vi "Main.vi"(7 "sweep rate, /min":dbl=0.2, 8 "sweep to:":dbl=-0.5, 9 "sweep":T6(radio)=enum."time_sweep") -> ()   [LabVIEW 2017] (continued)
                      n3711 = Number To Decimal String(number=w4969) -> (decimal integer string=w4968:string)  [unwired: 1 in]
                      n3712 = GPIB Write(0:w4968, 1:"OUTP?2") -> (6:w4974:errorcluster)  [unwired: 3 in, 1 out]
                      n3713 = GPIB Read(0:w4968, 1:3200, 3:w4974) -> (5:w4972:string)  [unwired: 2 in, 2 out]
                      n3714 = Fract/Exp String To Number(string=w4972) -> (number=w4971:dbl)  [unwired: 3 in, 1 out]
                      n3715 = Build Array (concatenate)(w4976, w4971) -> (w4975:dbl[])
                    }
                  }
                  n3716 = property on="data" class="Arr (strict)"("Value"=w4966) -> ()  [unwired: 2 in, 2 out]
                }
                frame #10 {
                  # "check if in-phase\nsignal on lock-in 6 \nis to be measured"
                  n3717 = property on="data" class="Arr (strict)"() -> ("Value"=w4978:dbl[])  [unwired: 2 in, 2 out]
                  n3718 = local read "SR830_6_ip"() -> (w4977:bool)
                  n3719 = case shown="True" w4977 {
                    tunnel: w4978 -> [w4980 w4989]
                    tunnel: [w4980 w4988] -> w4979
                    frame False {
                      # "we are not measuring in phase signal on lock-in 6 (SR830_6_ip)"
                    }
                    frame True {
                      # "we are  measuring lock-in 6 in phase (SR830_6_ip)"
                      n3720 = local read "SR830_6"() -> (w4982:u8)
                      n3721 = Number To Decimal String(number=w4982) -> (decimal integer string=w4981:string)  [unwired: 1 in]
                      n3722 = GPIB Write(0:w4981, 1:"OUTR?1") -> (6:w4987:errorcluster)  [unwired: 3 in, 1 out]
                      n3723 = GPIB Read(0:w4981, 1:3200, 3:w4987) -> (5:w4985:string)  [unwired: 2 in, 2 out]
                      n3724 = Fract/Exp String To Number(string=w4985) -> (number=w4984:dbl)  [unwired: 3 in, 1 out]
                      n3725 = Build Array (concatenate)(w4989, w4984) -> (w4988:dbl[])
                    }
                  }
                  n3726 = property on="data" class="Arr (strict)"("Value"=w4979) -> ()  [unwired: 2 in, 2 out]
                }
                frame #11 {
                  # "check if out-of-phase\nsignal on lock-in 6 \nis to be measured"
                  n3727 = property on="data" class="Arr (strict)"() -> ("Value"=w4991:dbl[])  [unwired: 2 in, 2 out]
                  n3728 = local read "SR830_6_oop"() -> (w4990:bool)
                  n3729 = case shown="True" w4990 {
                    tunnel: w4991 -> [w4993 w5002]
                    tunnel: [w4993 w5001] -> w4992
                    frame False {
                      # "we are not measuring out of phase signal on lock-in 6 (SR830_6_oop)"
                    }
                    frame True {
                      # "we are  measuring lock-in 6, out of phase (SR830_6_oop)"
                      n3730 = local read "SR830_6"() -> (w4995:u8)
                      n3731 = Number To Decimal String(number=w4995) -> (decimal integer string=w4994:string)  [unwired: 1 in]
                      n3732 = GPIB Write(0:w4994, 1:"OUTR?2") -> (6:w5000:errorcluster)  [unwired: 3 in, 1 out]
                      n3733 = GPIB Read(0:w4994, 1:3200, 3:w5000) -> (5:w4998:string)  [unwired: 2 in, 2 out]
                      n3734 = Fract/Exp String To Number(string=w4998) -> (number=w4997:dbl)  [unwired: 3 in, 1 out]
                      n3735 = Build Array (concatenate)(w5002, w4997) -> (w5001:dbl[])
                    }
                  }
                  n3736 = property on="data" class="Arr (strict)"("Value"=w4992) -> ()  [unwired: 2 in, 2 out]
                }
                frame #12 {
                  # "check if in-phase\nsignal on lock-in 7 \nis to be measured"
                  n3737 = property on="data" class="Arr (strict)"() -> ("Value"=w5004:dbl[])  [unwired: 2 in, 2 out]
                  n3738 = local read "SR830_7_ip"() -> (w5003:bool)
                  n3739 = case shown="True" w5003 {
                    tunnel: w5004 -> [w5006 w5015]
                    tunnel: [w5006 w5014] -> w5005
                    frame False {
                    }
                    frame True {
                      # "we are  measuring lock-in 7 in phase (SR830_7_ip)"
                      n3740 = local read "SR830_7"() -> (w5008:u8)
                      n3741 = Number To Decimal String(number=w5008) -> (decimal integer string=w5007:string)  [unwired: 1 in]
                      n3742 = GPIB Write(0:w5007, 1:"OUTR?1") -> (6:w5013:errorcluster)  [unwired: 3 in, 1 out]
                      n3743 = GPIB Read(0:w5007, 1:3200, 3:w5013) -> (5:w5011:string)  [unwired: 2 in, 2 out]
                      n3744 = Fract/Exp String To Number(string=w5011) -> (number=w5010:dbl)  [unwired: 3 in, 1 out]
                      n3745 = Build Array (concatenate)(w5015, w5010) -> (w5014:dbl[])
                    }
                  }
                  n3746 = property on="data" class="Arr (strict)"("Value"=w5005) -> ()  [unwired: 2 in, 2 out]
                }
                frame #13 {
                  # "check if out-of-phase\nsignal on lock-in 7 \nis to be measured"
                  n3747 = property on="data" class="Arr (strict)"() -> ("Value"=w5017:dbl[])  [unwired: 2 in, 2 out]
                  n3748 = local read "SR830_7_oop"() -> (w5016:bool)
                  n3749 = case shown="True" w5016 {
                    tunnel: w5017 -> [w5019 w5028]
                    tunnel: [w5019 w5027] -> w5018
                    frame False {
                    }
                    frame True {
                      # "we are  measuring lock-in 7 out of phase (SR830_7_oop)"
                      n3750 = local read "SR830_7"() -> (w5021:u8)
                      n3751 = Number To Decimal String(number=w5021) -> (decimal integer string=w5020:string)  [unwired: 1 in]
                      n3752 = GPIB Write(0:w5020, 1:"OUTR?2") -> (6:w5026:errorcluster)  [unwired: 3 in, 1 out]
                      n3753 = GPIB Read(0:w5020, 1:3200, 3:w5026) -> (5:w5024:string)  [unwired: 2 in, 2 out]
                      n3754 = Fract/Exp String To Number(string=w5024) -> (number=w5023:dbl)  [unwired: 3 in, 1 out]
                      n3755 = Build Array (concatenate)(w5028, w5023) -> (w5027:dbl[])
                    }
                  }
                  n3756 = property on="data" class="Arr (strict)"("Value"=w5018) -> ()  [unwired: 2 in, 2 out]
                }
                frame #14 {
                  # "check if in-phase\nsignal on lock-in 8 \nis to be measured"
                  n3757 = property on="data" class="Arr (strict)"() -> ("Value"=w5030:dbl[])  [unwired: 2 in, 2 out]
                  n3758 = local read "SR830_8_ip"() -> (w5029:bool)
                  n3759 = case shown="True" w5029 {
                    tunnel: w5030 -> [w5032 w5041]
                    tunnel: [w5032 w5040] -> w5031
                    frame False {
                    }
                    frame True {
                      # "we are  measuring lock-in 8 in phase (SR830_8_ip)"
                      n3760 = local read "SR830_8"() -> (w5034:u8)
                      n3761 = Number To Decimal String(number=w5034) -> (decimal integer string=w5033:string)  [unwired: 1 in]
                      n3762 = GPIB Write(0:w5033, 1:"OUTR?1") -> (6:w5039:errorcluster)  [unwired: 3 in, 1 out]
                      n3763 = GPIB Read(0:w5033, 1:3200, 3:w5039) -> (5:w5037:string)  [unwired: 2 in, 2 out]
                      n3764 = Fract/Exp String To Number(string=w5037) -> (number=w5036:dbl)  [unwired: 3 in, 1 out]
                      n3765 = Build Array (concatenate)(w5041, w5036) -> (w5040:dbl[])
                    }
                  }
                  n3766 = property on="data" class="Arr (strict)"("Value"=w5031) -> ()  [unwired: 2 in, 2 out]
                }
                frame #15 {
                  # "check if out-of-phase\nsignal on lock-in 8 \nis to be measured"
                  n3767 = property on="data" class="Arr (strict)"() -> ("Value"=w5043:dbl[])  [unwired: 2 in, 2 out]
                  n3768 = local read "SR830_8_oop"() -> (w5042:bool)
                  n3769 = case shown="True" w5042 {
                    tunnel: w5043 -> [w5045 w5054]
                    tunnel: [w5045 w5053] -> w5044
                    frame False {
                    }
                    frame True {
                      # "we are  measuring lock-in 8 out of phase (SR830_8_oop)"
                      n3770 = local read "SR830_8"() -> (w5047:u8)
                      n3771 = Number To Decimal String(number=w5047) -> (decimal integer string=w5046:string)  [unwired: 1 in]
                      n3772 = GPIB Write(0:w5046, 1:"OUTR?2") -> (6:w5052:errorcluster)  [unwired: 3 in, 1 out]
                      n3773 = GPIB Read(0:w5046, 1:3200, 3:w5052) -> (5:w5050:string)  [unwired: 2 in, 2 out]
                      n3774 = Fract/Exp String To Number(string=w5050) -> (number=w5049:dbl)  [unwired: 3 in, 1 out]
                      n3775 = Build Array (concatenate)(w5054, w5049) -> (w5053:dbl[])
                    }
                  }
                  n3776 = property on="data" class="Arr (strict)"("Value"=w5044) -> ()  [unwired: 2 in, 2 out]
                }
                frame #16 {
                  # "Measure MFLI_V if \nit is checked"
                  n3777 = property on="MFLI_V1" class="Bool (strict)"() -> ("Value"=w5055:bool)  [unwired: 2 in, 2 out]
                  n3778 = property on="data" class="Arr (strict)"() -> ("Value"=w5057:dbl[])  [unwired: 2 in, 2 out]
                  n3779 = case shown="True" w5055 {
                    tunnel: w5057 -> [w5058 w5063]
                    tunnel: [w5058 w5062] -> w5056
                    frame False {
                      # "We are not recording Step Value if it is linetrace"
                    }
                    frame True {
                      n3780 = flat-sequence {
                        tunnel: [w5067] -> w5061
                        tunnel: [w5066] -> w5060
                        tunnel: [w5065] -> w5059
                        frame #0 {
                          n3781 = property on="HandleOut" class="Clust (strict)"() -> ("Value"=w5069:T5)  [unwired: 2 in, 2 out]
                          n3782 = call "MFLIcontrol.vi"("MFLI function"=MFLIcommand."measure XY on demod0", "handle in"=w5069) -> ("Demod Sample Out 2"=w5064:T22)  [unwired: 6 in, 3 out]
                          n3783 = Unbundle(w5064) -> ("X (Vrms)"=w5067:dbl, "Y (Vrms)"=w5066:dbl, "Freq (Hz)"=w5065:dbl)  [unwired: 6 out]
                        }
                      }
                      n3784 = Build Array (concatenate)(w5063, w5061, w5060, w5059) -> (w5062:dbl[])
                    }
                  }
                  n3785 = property on="data" class="Arr (strict)"("Value"=w5056) -> ()  [unwired: 2 in, 2 out]
                }
                frame #17 {
                  # "Measure MFLI_I if \nit is checked"
                  n3786 = property on="MFLI_I1" class="Bool (strict)"() -> ("Value"=w5070:bool)  [unwired: 2 in, 2 out]
                  n3787 = property on="data" class="Arr (strict)"() -> ("Value"=w5072:dbl[])  [unwired: 2 in, 2 out]
                  n3788 = case shown="True" w5070 {
                    tunnel: w5072 -> [w5073 w5078]
                    tunnel: [w5073 w5077] -> w5071
                    frame False {
                      # "We are not recording Step Value if it is linetrace"
                    }
                    frame True {
                      n3789 = flat-sequence {
                        tunnel: [w5081] -> w5076
                        tunnel: [w5080] -> w5075
                        tunnel: [w5079] -> w5074
                        frame #0 {
                          n3790 = property on="HandleOut" class="Clust (strict)"() -> ("Value"=w5084:T5)  [unwired: 2 in, 2 out]
                          n3791 = call "MFLIcontrol.vi"("MFLI function"=MFLIcommand."measure current", "handle in"=w5084) -> ("Demod Sample Out 3"=w5082:T22)  [unwired: 6 in, 3 out]
                          n3792 = Unbundle(w5082) -> ("X (Vrms)"=w5081:dbl, "Y (Vrms)"=w5080:dbl, "Freq (Hz)"=w5079:dbl)  [unwired: 6 out]
                        }
                      }
                      n3793 = Build Array (concatenate)(w5078, w5076, w5075, w5074) -> (w5077:dbl[])
                    }
                  }
                  n3794 = property on="data" class="Arr (strict)"("Value"=w5071) -> ()  [unwired: 2 in, 2 out]
                }
                frame #18 {
                  # "Measure MFLI_V if \nit is checked"
                  n3795 = local read "MFLI_V2"() -> (w5085:bool)
                  n3796 = property on="data" class="Arr (strict)"() -> ("Value"=w5087:dbl[])  [unwired: 2 in, 2 out]
                  n3797 = case shown="True" w5085 {
                    tunnel: w5087 -> [w5088 w5093]
                    tunnel: [w5088 w5092] -> w5086
                    frame False {
                    }
                    frame True {
                      n3798 = flat-sequence {
                        tunnel: [w5098] -> w5091
                        tunnel: [w5097] -> w5090
                        tunnel: [w5096] -> w5089
                        frame #0 {
                          n3799 = property on="Handle Out 2" class="Clust (strict)"() -> ("Value"=w5094:T5)  [unwired: 2 in, 2 out]
                          n3800 = call "MFLIcontrol.vi"("MFLI function"=MFLIcommand."measure XY on demod0", "handle in"=w5094) -> ("Demod Sample Out 2"=w5095:T22)  [unwired: 6 in, 3 out]
                          n3801 = Unbundle(w5095) -> ("X (Vrms)"=w5098:dbl, "Y (Vrms)"=w5097:dbl, "Freq (Hz)"=w5096:dbl)  [unwired: 6 out]
                        }
                      }
                      n3802 = Build Array (concatenate)(w5093, w5091, w5090, w5089) -> (w5092:dbl[])
                    }
                  }
                  n3803 = property on="data" class="Arr (strict)"("Value"=w5086) -> ()  [unwired: 2 in, 2 out]
                }
                frame #19 {
                  # "Measure MFLI_I if \nit is checked"
                  n3804 = local read "MFLI_I2"() -> (w5100:bool)
                  n3805 = property on="data" class="Arr (strict)"() -> ("Value"=w5102:dbl[])  [unwired: 2 in, 2 out]
                  n3806 = case shown="True" w5100 {
                    tunnel: w5102 -> [w5103 w5108]
                    tunnel: [w5103 w5107] -> w5101
                    frame False {
                    }
                    frame True {
                      n3807 = flat-sequence {
                        tunnel: [w5113] -> w5106
                        tunnel: [w5112] -> w5105
                        tunnel: [w5111] -> w5104
                        frame #0 {
                          n3808 = property on="Handle Out 2" class="Clust (strict)"() -> ("Value"=w5110:T5)  [unwired: 2 in, 2 out]
                          n3809 = call "MFLIcontrol.vi"("MFLI function"=MFLIcommand."measure current", "handle in"=w5110) -> ("Demod Sample Out 3"=w5109:T22)  [unwired: 6 in, 3 out]
                          n3810 = Unbundle(w5109) -> ("X (Vrms)"=w5113:dbl, "Y (Vrms)"=w5112:dbl, "Freq (Hz)"=w5111:dbl)  [unwired: 6 out]
                        }
                      }
                      n3811 = Build Array (concatenate)(w5108, w5106, w5105, w5104) -> (w5107:dbl[])
                    }
                  }
                  n3812 = property on="data" class="Arr (strict)"("Value"=w5101) -> ()  [unwired: 2 in, 2 out]
                }
                frame #20 {
                  # "check if voltage \non 2400 SouceMeter 1\nis to be measured"
                  n3813 = property on="data" class="Arr (strict)"() -> ("Value"=w5116:dbl[])  [unwired: 2 in, 2 out]
                  n3814 = local read "2400 1 meas v"() -> (w5115:bool)
                  n3815 = case shown="True" w5115 {
                    tunnel: w5116 -> [w5118 w5129]
                    tunnel: [w5118 w5128] -> w5117
                    frame False {
                      # "we are not measuring 2400 1, voltage (2400_1_v)"
                    }
                    frame True {
                      # "we are  measuring 2400 1, voltage (2400_1_v)"
                      n3816 = local read "2400 1 addr"() -> (w5123:u8)
                      n3817 = Number To Decimal String(number=w5123) -> (decimal integer string=w5122:string)  [unwired: 1 in]
                      n3818 = GPIB Write(0:w5122, 1:":READ?") -> (6:w5127:errorcluster)  [unwired: 3 in, 1 out]
                      n3819 = GPIB Read(0:w5122, 1:3200, 3:w5127) -> (5:w5120:string)  [unwired: 2 in, 2 out]
                      n3820 = String Subset(string=w5120, length (rest)=13) -> (substring=w5119:string)  [unwired: 1 in]
                      n3821 = Fract/Exp String To Number(string=w5119) -> (number=w5125:dbl)  [unwired: 3 in, 1 out]
                      n3822 = Build Array (concatenate)(w5129, w5125) -> (w5128:dbl[])
                    }
                  }
                  n3823 = property on="data" class="Arr (strict)"("Value"=w5117) -> ()  [unwired: 2 in, 2 out]
                }
                frame #21 {
                  # "check if current \non 2400 SouceMeter 1\nis to be measured"
                  n3824 = property on="data" class="Arr (strict)"() -> ("Value"=w5131:dbl[])  [unwired: 2 in, 2 out]
                  n3825 = local read "2400 1 meas i"() -> (w5130:bool)
                  n3826 = case shown="True" w5130 {
                    tunnel: w5131 -> [w5133 w5145]
                    tunnel: [w5133 w5144] -> w5132
                    frame False {
                      # "we are not measuring 2400 1, current (2400_1_i)"
                    }
                    frame True {
                      # "we are  measuring 2400 1, current (2400_1_i)"
                      n3827 = local read "2400 1 addr"() -> (w5139:u8)
                      n3828 = Number To Decimal String(number=w5139) -> (decimal integer string=w5138:string)  [unwired: 1 in]
                      n3829 = GPIB Write(0:w5138, 1:":READ?") -> (6:w5143:errorcluster)  [unwired: 3 in, 1 out]
                      n3830 = GPIB Read(0:w5138, 1:3200, 3:w5143) -> (5:w5136:string)  [unwired: 2 in, 2 out]
                      n3831 = String Subset(string=w5136, offset (0)=14, length (rest)=13) -> (substring=w5135:string)
                      n3832 = Fract/Exp String To Number(string=w5135) -> (number=w5141:dbl)  [unwired: 3 in, 1 out]
                      n3833 = Build Array (concatenate)(w5145, w5141) -> (w5144:dbl[])
                    }
                  }
                  n3834 = property on="data" class="Arr (strict)"("Value"=w5132) -> ()  [unwired: 2 in, 2 out]
                }
                frame #22 {
                  # "check if voltage \non 2400 SouceMeter 2\nis to be measured"
                  n3835 = property on="data" class="Arr (strict)"() -> ("Value"=w5147:dbl[])  [unwired: 2 in, 2 out]
                  n3836 = local read "2400 2 meas v"() -> (w5146:bool)
                  n3837 = case shown="True" w5146 {
                    tunnel: w5147 -> [w5149 w5160]
                    tunnel: [w5149 w5159] -> w5148
                    frame False {
                      # "we are not measuring 2400 2, voltage (2400_2_v)"
                    }
                    frame True {
                      # "we are  measuring 2400 2, voltage (2400_2_v)"
                      n3838 = local read "2400 2 addr"() -> (w5154:u8)
                      n3839 = Number To Decimal String(number=w5154) -> (decimal integer string=w5153:string)  [unwired: 1 in]
                      n3840 = GPIB Write(0:w5153, 1:":READ?") -> (6:w5158:errorcluster)  [unwired: 3 in, 1 out]
                      n3841 = GPIB Read(0:w5153, 1:3200, 3:w5158) -> (5:w5151:string)  [unwired: 2 in, 2 out]
                      n3842 = String Subset(string=w5151, length (rest)=13) -> (substring=w5150:string)  [unwired: 1 in]
                      n3843 = Fract/Exp String To Number(string=w5150) -> (number=w5156:dbl)  [unwired: 3 in, 1 out]
                      n3844 = Build Array (concatenate)(w5160, w5156) -> (w5159:dbl[])
                    }
                  }
                  n3845 = property on="data" class="Arr (strict)"("Value"=w5148) -> ()  [unwired: 2 in, 2 out]
                }
                frame #23 {
                  # "check if current \non 2400 SouceMeter 2\nis to be measured"
                  n3846 = property on="data" class="Arr (strict)"() -> ("Value"=w5162:dbl[])  [unwired: 2 in, 2 out]
                  n3847 = local read "2400 2 meas i"() -> (w5161:bool)
                  n3848 = case shown="True" w5161 {
                    tunnel: w5162 -> [w5164 w5176]
                    tunnel: [w5164 w5175] -> w5163
                    frame False {
                      # "we are not measuring 2400 2, current (2400_2_i)"
                    }
                    frame True {
                      # "we are  measuring 2400 2, current (2400_2_i)"
                      n3849 = local read "2400 2 addr"() -> (w5170:u8)
                      n3850 = Number To Decimal String(number=w5170) -> (decimal integer string=w5169:string)  [unwired: 1 in]
                      n3851 = GPIB Write(0:w5169, 1:":READ?") -> (6:w5174:errorcluster)  [unwired: 3 in, 1 out]
                      n3852 = GPIB Read(0:w5169, 1:3200, 3:w5174) -> (5:w5167:string)  [unwired: 2 in, 2 out]
                      n3853 = String Subset(string=w5167, offset (0)=14, length (rest)=13) -> (substring=w5166:string)
                      n3854 = Fract/Exp String To Number(string=w5166) -> (number=w5172:dbl)  [unwired: 3 in, 1 out]
                      n3855 = Build Array (concatenate)(w5176, w5172) -> (w5175:dbl[])
                    }
                  }
                  n3856 = property on="data" class="Arr (strict)"("Value"=w5163) -> ()  [unwired: 2 in, 2 out]
                }
                frame #24 {
                  # "check if voltage \non 2400 SouceMeter 3\nis to be measured"
                  n3857 = property on="data" class="Arr (strict)"() -> ("Value"=w5178:dbl[])  [unwired: 2 in, 2 out]
                  n3858 = local read "2400 3 meas v"() -> (w5177:bool)
                  n3859 = case shown="True" w5177 {
                    tunnel: w5178 -> [w5180 w5191]
                    tunnel: [w5180 w5190] -> w5179
                    frame False {
                      # "we are not measuring 2400 3, voltage (2400_3_v)"
                    }
                    frame True {
                      # "we are  measuring 2400 3, voltage (2400_3_v)"
                      n3860 = local read "2400 3 addr"() -> (w5185:u8)
                      n3861 = Number To Decimal String(number=w5185) -> (decimal integer string=w5184:string)  [unwired: 1 in]
                      n3862 = GPIB Write(0:w5184, 1:":READ?") -> (6:w5189:errorcluster)  [unwired: 3 in, 1 out]
                      n3863 = GPIB Read(0:w5184, 1:3200, 3:w5189) -> (5:w5182:string)  [unwired: 2 in, 2 out]
                      n3864 = String Subset(string=w5182, length (rest)=13) -> (substring=w5181:string)  [unwired: 1 in]
                      n3865 = Fract/Exp String To Number(string=w5181) -> (number=w5187:dbl)  [unwired: 3 in, 1 out]
                      n3866 = Build Array (concatenate)(w5191, w5187) -> (w5190:dbl[])
                    }
                  }
                  n3867 = property on="data" class="Arr (strict)"("Value"=w5179) -> ()  [unwired: 2 in, 2 out]
                }
                frame #25 {
                  # "check if current \non 2400 SouceMeter 3\nis to be measured"
                  n3868 = property on="data" class="Arr (strict)"() -> ("Value"=w5193:dbl[])  [unwired: 2 in, 2 out]
                  n3869 = local read "2400 3 meas i"() -> (w5192:bool)
                  n3870 = case shown="True" w5192 {
                    tunnel: w5193 -> [w5195 w5207]
                    tunnel: [w5195 w5206] -> w5194
                    frame False {
                      # "we are not measuring 2400 3, current (2400_3_i)"
                    }
                    frame True {
                      # "we are  measuring 2400 3, current (2400_3_i)"
                      n3871 = local read "2400 3 addr"() -> (w5201:u8)
                      n3872 = Number To Decimal String(number=w5201) -> (decimal integer string=w5200:string)  [unwired: 1 in]
                      n3873 = GPIB Write(0:w5200, 1:":READ?") -> (6:w5205:errorcluster)  [unwired: 3 in, 1 out]
                      n3874 = GPIB Read(0:w5200, 1:3200, 3:w5205) -> (5:w5198:string)  [unwired: 2 in, 2 out]
                      n3875 = String Subset(string=w5198, offset (0)=14, length (rest)=13) -> (substring=w5197:string)
                      n3876 = Fract/Exp String To Number(string=w5197) -> (number=w5203:dbl)  [unwired: 3 in, 1 out]
                      n3877 = Build Array (concatenate)(w5207, w5203) -> (w5206:dbl[])
                    }
                  }
                  n3878 = property on="data" class="Arr (strict)"("Value"=w5194) -> ()  [unwired: 2 in, 2 out]
                }
                frame #26 {
                  # "check if 1st channel \non Keithley 2182A 1\nis to be measured"
                  n3879 = property on="data" class="Arr (strict)"() -> ("Value"=w5209:dbl[])  [unwired: 2 in, 2 out]
                  n3880 = local read "2182A 1 ch1"() -> (w5208:bool)
                  n3881 = case shown="True" w5208 {
                    tunnel: w5209 -> [w5211 w5220]
                    tunnel: [w5211 w5219] -> w5210
                    frame False {
                      # "we are not measuring 2182A 1 channel 1 (2182A_1_ch1)"
                    }
                    frame True {
                      # "we are  measuring 2182A 1 channel 1 (2182A_1_ch1)"
                      n3882 = local read "2182A 1 addr"() -> (w5214:u8)
                      n3883 = Number To Decimal String(number=w5214) -> (decimal integer string=w5213:string)  [unwired: 1 in]
                      n3884 = GPIB Write(0:w5213, 1:":SENSe:DATA:FRES?") -> (6:w5218:errorcluster)  [unwired: 3 in, 1 out]
                      n3885 = GPIB Read(0:w5213, 1:200, 3:w5218) -> (5:w5212:string)  [unwired: 2 in, 2 out]
                      n3886 = Fract/Exp String To Number(string=w5212) -> (number=w5216:dbl)  [unwired: 3 in, 1 out]
                      n3887 = Build Array (concatenate)(w5220, w5216) -> (w5219:dbl[])
                    }
                  }
                  n3888 = property on="data" class="Arr (strict)"("Value"=w5210) -> ()  [unwired: 2 in, 2 out]
                }
                frame #27 {
                  # "check if 2nd channel \non Keithley 2182A 1\nis to be measured"
                  n3889 = property on="data" class="Arr (strict)"() -> ("Value"=w5222:dbl[])  [unwired: 2 in, 2 out]
                  n3890 = local read "2182A 1 ch2"() -> (w5221:bool)
                  n3891 = case shown="True" w5221 {
                    tunnel: w5222 -> [w5224 w5237]
                    tunnel: [w5224 w5236] -> w5223
                    frame False {
                      # "we are not measuring 2182A 1 channel 2 (2182A_1_ch2)"
                    }
                    frame True {
                      # "switching to channel 2 and then\nback to channel 1"
                      # "we are  measuring 2182A 1 channel 2 (2182A_1_ch2)"
                      n3892 = local read "2182A 1 addr"() -> (w5231:u8)
                      n3893 = Number To Decimal String(number=w5231) -> (decimal integer string=w5226:string)  [unwired: 1 in]
                      n3894 = GPIB Write(0:w5226, 1:":SENSe:CHAN 2") -> (6:w5228:errorcluster)  [unwired: 3 in, 1 out]
                      n3895 = GPIB Write(0:w5226, 1:":SENSe:DATA:FRES?", 3:w5228) -> (6:w5235:errorcluster)  [unwired: 2 in, 1 out]
                      n3896 = GPIB Read(0:w5226, 1:200, 3:w5235) -> (5:w5230:string, 7:w5227:errorcluster)  [unwired: 2 in, 1 out]
                      n3897 = GPIB Write(0:w5226, 1:":SENSe:CHAN 1", 3:w5227) -> ()  [unwired: 2 in, 2 out]
                      n3898 = Fract/Exp String To Number(string=w5230) -> (number=w5233:dbl)  [unwired: 3 in, 1 out]
                      n3899 = Build Array (concatenate)(w5237, w5233) -> (w5236:dbl[])
                    }
                  }
                  n3900 = property on="data" class="Arr (strict)"("Value"=w5223) -> ()  [unwired: 2 in, 2 out]
                }
                frame #28 {
                  # "check if 1st channel \non Keithley 2182A 2\nis to be measured"
                  n3901 = property on="data" class="Arr (strict)"() -> ("Value"=w5239:dbl[])  [unwired: 2 in, 2 out]
                  n3902 = local read "2182A 2 ch1"() -> (w5238:bool)
                  n3903 = case shown="True" w5238 {
                    tunnel: w5239 -> [w5241 w5250]
                    tunnel: [w5241 w5249] -> w5240
                    frame False {
                      # "we are not measuring 2182A 2 channel 1 (2182A_2_ch1)"
                    }
                    frame True {
                      # "we are  measuring 2182A 2 channel 1 (2182A_2_ch1)"
                      n3904 = local read "2182A 2 addr"() -> (w5244:u8)
                      n3905 = Number To Decimal String(number=w5244) -> (decimal integer string=w5243:string)  [unwired: 1 in]
                      n3906 = GPIB Write(0:w5243, 1:":SENSe:DATA:FRES?") -> (6:w5248:errorcluster)  [unwired: 3 in, 1 out]
                      n3907 = GPIB Read(0:w5243, 1:200, 3:w5248) -> (5:w5242:string)  [unwired: 2 in, 2 out]
                      n3908 = Fract/Exp String To Number(string=w5242) -> (number=w5246:dbl)  [unwired: 3 in, 1 out]
                      n3909 = Build Array (concatenate)(w5250, w5246) -> (w5249:dbl[])
                    }
                  }
                  n3910 = property on="data" class="Arr (strict)"("Value"=w5240) -> ()  [unwired: 2 in, 2 out]
                }
                frame #29 {
                  # "check if 2nd channel \non Keithley 2182A 2\nis to be measured"
                  n3911 = property on="data" class="Arr (strict)"() -> ("Value"=w5252:dbl[])  [unwired: 2 in, 2 out]
                  n3912 = local read "2182A 2 ch2"() -> (w5251:bool)
                  n3913 = case shown="True" w5251 {
                    tunnel: w5252 -> [w5254 w5267]
                    tunnel: [w5254 w5266] -> w5253
                    frame False {
                      # "we are not measuring 2182A 2 channel 2 (2182A_2_ch2)"
                    }
                    frame True {
                      # "switching to channel 2 and then\nback to channel 1"
                      # "we are  measuring 2182A 2 channel 2 (2182A_2_ch2)"
                      n3914 = local read "2182A 2 addr"() -> (w5261:u8)
                      n3915 = Number To Decimal String(number=w5261) -> (decimal integer string=w5256:string)  [unwired: 1 in]
                      n3916 = GPIB Write(0:w5256, 1:":SENSe:CHAN 2") -> (6:w5258:errorcluster)  [unwired: 3 in, 1 out]
                      n3917 = GPIB Write(0:w5256, 1:":SENSe:DATA:FRES?", 3:w5258) -> (6:w5265:errorcluster)  [unwired: 2 in, 1 out]
                      n3918 = GPIB Read(0:w5256, 1:200, 3:w5265) -> (5:w5260:string, 7:w5257:errorcluster)  [unwired: 2 in, 1 out]
                      n3919 = GPIB Write(0:w5256, 1:":SENSe:CHAN 1", 3:w5257) -> ()  [unwired: 2 in, 2 out]
                      n3920 = Fract/Exp String To Number(string=w5260) -> (number=w5263:dbl)  [unwired: 3 in, 1 out]
                      n3921 = Build Array (concatenate)(w5267, w5263) -> (w5266:dbl[])
                    }
                  }
                  n3922 = property on="data" class="Arr (strict)"("Value"=w5253) -> ()  [unwired: 2 in, 2 out]
                }
                frame #30 {
                  # "check if 1st channel \non Keithley 2182A 3\nis to be measured"
                  n3923 = property on="data" class="Arr (strict)"() -> ("Value"=w5269:dbl[])  [unwired: 2 in, 2 out]
                  n3924 = local read "2182A 3 ch1"() -> (w5268:bool)
                  n3925 = case shown="True" w5268 {
                    tunnel: w5269 -> [w5271 w5280]
                    tunnel: [w5271 w5279] -> w5270
                    frame False {
                      # "we are not measuring 2182A 3 channel 1 (2182A_3_ch1)"
                    }
                    frame True {
                      # "we are  measuring 2182A 3 channel 1 (2182A_3_ch1)"
                      n3926 = local read "2182A 3 addr"() -> (w5274:u8)
                      n3927 = Number To Decimal String(number=w5274) -> (decimal integer string=w5273:string)  [unwired: 1 in]
                      n3928 = GPIB Write(0:w5273, 1:":SENSe:DATA:FRES?") -> (6:w5278:errorcluster)  [unwired: 3 in, 1 out]
                      n3929 = GPIB Read(0:w5273, 1:200, 3:w5278) -> (5:w5272:string)  [unwired: 2 in, 2 out]
                      n3930 = Fract/Exp String To Number(string=w5272) -> (number=w5276:dbl)  [unwired: 3 in, 1 out]
                      n3931 = Build Array (concatenate)(w5280, w5276) -> (w5279:dbl[])
                    }
                  }
                  n3932 = property on="data" class="Arr (strict)"("Value"=w5270) -> ()  [unwired: 2 in, 2 out]
                }
                frame #31 {
                  # "check if 2nd channel \non Keithley 2182A 3\nis to be measured"
                  n3933 = property on="data" class="Arr (strict)"() -> ("Value"=w5282:dbl[])  [unwired: 2 in, 2 out]
                  n3934 = local read "2182A 3 ch2"() -> (w5281:bool)
                  n3935 = case shown="True" w5281 {
                    tunnel: w5282 -> [w5284 w5297]
                    tunnel: [w5284 w5296] -> w5283
                    frame False {
                      # "we are not measuring 2182A 3 channel 2 (2182A_3_ch2)"
                    }
                    frame True {
                      # "switching to channel 2 and then\nback to channel 1"
                      # "we are  measuring 2182A 3 channel 2 (2182A_3_ch2)"
                      n3936 = local read "2182A 3 addr"() -> (w5291:u8)
                      n3937 = Number To Decimal String(number=w5291) -> (decimal integer string=w5286:string)  [unwired: 1 in]
                      n3938 = GPIB Write(0:w5286, 1:":SENSe:CHAN 2") -> (6:w5288:errorcluster)  [unwired: 3 in, 1 out]
                      n3939 = GPIB Write(0:w5286, 1:":SENSe:DATA:FRES?", 3:w5288) -> (6:w5295:errorcluster)  [unwired: 2 in, 1 out]
                      n3940 = GPIB Read(0:w5286, 1:200, 3:w5295) -> (5:w5290:string, 7:w5287:errorcluster)  [unwired: 2 in, 1 out]
                      n3941 = GPIB Write(0:w5286, 1:":SENSe:CHAN 1", 3:w5287) -> ()  [unwired: 2 in, 2 out]
                      n3942 = Fract/Exp String To Number(string=w5290) -> (number=w5293:dbl)  [unwired: 3 in, 1 out]
                      n3943 = Build Array (concatenate)(w5297, w5293) -> (w5296:dbl[])
                    }
                  }
                  n3944 = property on="data" class="Arr (strict)"("Value"=w5283) -> ()  [unwired: 2 in, 2 out]
                }
                frame #32 {
                  # "check if 1st channel \non Keithley 2182A 4\nis to be measured"
                  n3945 = property on="data" class="Arr (strict)"() -> ("Value"=w5299:dbl[])  [unwired: 2 in, 2 out]
                  n3946 = local read "2182A 4 ch1"() -> (w5298:bool)
                  n3947 = case shown="True" w5298 {
                    tunnel: w5299 -> [w5301 w5310]
                    tunnel: [w5301 w5309] -> w5300
                    frame False {
                      # "we are not measuring 2182A 4 channel 1 (2182A_4_ch1)"
                    }
                    frame True {
                      # "we are  measuring 2182A 4 channel 1 (2182A_4_ch1)"
                      n3948 = local read "2182A 4 addr"() -> (w5304:u8)
                      n3949 = Number To Decimal String(number=w5304) -> (decimal integer string=w5303:string)  [unwired: 1 in]
                      n3950 = GPIB Write(0:w5303, 1:":SENSe:DATA:FRES?") -> (6:w5308:errorcluster)  [unwired: 3 in, 1 out]
                      n3951 = GPIB Read(0:w5303, 1:200, 3:w5308) -> (5:w5302:string)  [unwired: 2 in, 2 out]
                      n3952 = Fract/Exp String To Number(string=w5302) -> (number=w5306:dbl)  [unwired: 3 in, 1 out]
                      n3953 = Build Array (concatenate)(w5310, w5306) -> (w5309:dbl[])
                    }
                  }
                  n3954 = property on="data" class="Arr (strict)"("Value"=w5300) -> ()  [unwired: 2 in, 2 out]
                }
                frame #33 {
                  # "check if 2nd channel \non Keithley 2182A 4\nis to be measured"
                  n3955 = property on="data" class="Arr (strict)"() -> ("Value"=w5312:dbl[])  [unwired: 2 in, 2 out]
                  n3956 = local read "2182A 4 ch2"() -> (w5311:bool)
                  n3957 = case shown="False" w5311 {
                    tunnel: w5312 -> [w5314 w5327]
                    tunnel: [w5314 w5326] -> w5313
                    frame False {
                      # "we are not measuring 2182A 4 channel 2 (2182A_4_ch2)"
                    }
                    frame True {
                      # "switching to channel 2 and then\nback to channel 1"
                      # "we are  measuring 2182A 4 channel 2 (2182A_4_ch2)"
                      n3958 = local read "2182A 4 addr"() -> (w5321:u8)
                      n3959 = Number To Decimal String(number=w5321) -> (decimal integer string=w5316:string)  [unwired: 1 in]
                      n3960 = GPIB Write(0:w5316, 1:":SENSe:CHAN 2") -> (6:w5318:errorcluster)  [unwired: 3 in, 1 out]
                      n3961 = GPIB Write(0:w5316, 1:":SENSe:DATA:FRES?", 3:w5318) -> (6:w5325:errorcluster)  [unwired: 2 in, 1 out]
                      n3962 = GPIB Read(0:w5316, 1:200, 3:w5325) -> (5:w5320:string, 7:w5317:errorcluster)  [unwired: 2 in, 1 out]
                      n3963 = GPIB Write(0:w5316, 1:":SENSe:CHAN 1", 3:w5317) -> ()  [unwired: 2 in, 2 out]
                      n3964 = Fract/Exp String To Number(string=w5320) -> (number=w5323:dbl)  [unwired: 3 in, 1 out]
                      n3965 = Build Array (concatenate)(w5327, w5323) -> (w5326:dbl[])
                    }
                  }
                  n3966 = property on="data" class="Arr (strict)"("Value"=w5313) -> ()  [unwired: 2 in, 2 out]
                }
                frame #34 {
                  # "check if voltage on\nKeithley 2636A smua\nis to be measured"
                  n3967 = local read "2636A smua meas v"() -> (w5328:bool)
                  n3968 = property on="data" class="Arr (strict)"() -> ("Value"=w5329:dbl[])  [unwired: 2 in, 2 out]
                  n3969 = case shown="True" w5328 {
                    tunnel: w5329 -> [w5331 w5337]
                    tunnel: [w5331 w5336] -> w5330
                    frame False {
                      # "we are not measuring voltage on 2636A smua (2636A_smua_v)"
                    }
                    frame True {
                      # "we are  measuring voltage on 2636A smua (2636A_smua_v)"
                      n3970 = local read "2336A addr"() -> (w5332:refnum<visa-resource-name>)
                      n3971 = call "SinglePointMeasurement.vi"("Measure"=Measure."Voltage", "Channel"=Channel."a", "VISA resource name 2"=w5332) -> ("Measuremet"=w5334:dbl)  [unwired: 3 in, 4 out]
                      n3972 = Build Array (concatenate)(w5337, w5334) -> (w5336:dbl[])
                    }
                  }
                  n3973 = property on="data" class="Arr (strict)"("Value"=w5330) -> ()  [unwired: 2 in, 2 out]
                }
                frame #35 {
                  # "check if current on\nKeithley 2636A smua\nis to be measured"
                  n3974 = local read "2636A smua meas i"() -> (w5338:bool)
                  n3975 = property on="data" class="Arr (strict)"() -> ("Value"=w5339:dbl[])  [unwired: 2 in, 2 out]
                  n3976 = case shown="True" w5338 {
                    tunnel: w5339 -> [w5341 w5344]
                    tunnel: [w5341 w5343] -> w5340
                    frame False {
                      # "we are not measuring current on 2636A smua (2636A_smua_i)"
                    }
                    frame True {
                      # "we are  measuring current on 2636A smua (2636A_smua_i)"
                      n3977 = stacked-sequence {
                        tunnel: [_ w5353] -> w5342
                        frame #0 {
                          n3978 = local read "auto\nrange A"() -> (w5348:bool)
                          n3979 = local read "2336A addr"() -> (w5351:refnum<visa-resource-name>)
                          n3980 = Select(t="smua.AUTORANGE_ON", s=w5348, f="smua.AUTORANGE_OFF") -> (s? t:f=w5346:string)
                          n3981 = Concatenate Strings("smua.measure.autorangei = ", w5346) -> (w5345:string)
                          n3982 = VISA Write(VISA resource name=w5351, write buffer=w5345) -> ()  [unwired: 1 in, 3 out]
                        }
                        frame #1 {
                          n3983 = local read "2336A addr"() -> (w5355:refnum<visa-resource-name>)
                          n3984 = call "SinglePointMeasurement.vi"("Measure"=Measure."Current", "Channel"=Channel."a", "VISA resource name 2"=w5355) -> ("Measuremet"=w5353:dbl)  [unwired: 3 in, 4 out]
                        }
                      }
                      n3985 = Build Array (concatenate)(w5344, w5342) -> (w5343:dbl[])
                    }
                  }
                  n3986 = property on="data" class="Arr (strict)"("Value"=w5340) -> ()  [unwired: 2 in, 2 out]
                }
                frame #36 {
                  # "check if voltage on\nKeithley 2636A smub\nis to be measured"
                  n3987 = local read "2636A smub meas v"() -> (w5356:bool)
                  n3988 = property on="data" class="Arr (strict)"() -> ("Value"=w5357:dbl[])  [unwired: 2 in, 2 out]
                  n3989 = case shown="True" w5356 {
                    tunnel: w5357 -> [w5359 w5365]
                    tunnel: [w5359 w5364] -> w5358
                    frame False {
                      # "we are not measuring voltage on 2636A smub (2636A_smub_v)"
                    }
                    frame True {
                      # "we are  measuring voltage on 2636A smub (2636A_smub_v)"
                      n3990 = local read "2336A addr"() -> (w5363:refnum<visa-resource-name>)
                      n3991 = call "SinglePointMeasurement.vi"("Measure"=Measure."Voltage", "Channel"=Channel."b", "VISA resource name 2"=w5363) -> ("Measuremet"=w5361:dbl)  [unwired: 3 in, 4 out]
                      n3992 = Build Array (concatenate)(w5365, w5361) -> (w5364:dbl[])
                    }
                  }
                  n3993 = property on="data" class="Arr (strict)"("Value"=w5358) -> ()  [unwired: 2 in, 2 out]
                }
                frame #37 {
                  # "check if current on\nKeithley 2636A smub\nis to be measured"
                  n3994 = local read "2636A smub meas i"() -> (w5366:bool)
                  n3995 = property on="data" class="Arr (strict)"() -> ("Value"=w5367:dbl[])  [unwired: 2 in, 2 out]
                  n3996 = case shown="True" w5366 {
                    tunnel: w5367 -> [w5369 w5372]
                    tunnel: [w5369 w5371] -> w5368
                    frame False {
                      # "we are not measuring current on 2636A smub (2636A_smub_i)"
                    }
                    frame True {
                      # "we are  measuring current on 2636A smub (2636A_smub_i)"
                      n3997 = stacked-sequence {
                        tunnel: [_ w5381] -> w5370
                        frame #0 {
                          n3998 = local read "auto\nrange B"() -> (w5376:bool)
                          n3999 = local read "2336A addr"() -> (w5379:refnum<visa-resource-name>)
                          n4000 = Select(t="smub.AUTORANGE_ON", s=w5376, f="smub.AUTORANGE_OFF") -> (s? t:f=w5374:string)
                          n4001 = Concatenate Strings("smub.measure.autorangei = ", w5374) -> (w5373:string)
                          n4002 = VISA Write(VISA resource name=w5379, write buffer=w5373) -> ()  [unwired: 1 in, 3 out]
                        }
                        frame #1 {
                          n4003 = local read "2336A addr"() -> (w5383:refnum<visa-resource-name>)
                          n4004 = call "SinglePointMeasurement.vi"("Measure"=Measure."Current", "Channel"=Channel."b", "VISA resource name 2"=w5383) -> ("Measuremet"=w5381:dbl)  [unwired: 3 in, 4 out]
                        }
                      }
                      n4005 = Build Array (concatenate)(w5372, w5370) -> (w5371:dbl[])
                    }
                  }
                  n4006 = property on="data" class="Arr (strict)"("Value"=w5368) -> ()  [unwired: 2 in, 2 out]
                }
                frame #38 {
                  # "check if time\nis to be measured"
                  n4007 = property on="data" class="Arr (strict)"() -> ("Value"=w5386:dbl[])  [unwired: 2 in, 2 out]
                  n4008 = local read "measure time"() -> (w5385:bool)
                  n4009 = case shown="True" w5385 {
                    tunnel: w5386 -> [w5388 w5394]
                    tunnel: [w5388 w5393] -> w5387
                    tunnel: w5384 -> [_ w5391]
                    frame False {
                      # "we are not measuring time"
                    }
                    frame True {
                      # "seconds from the beginning of month"
                      # "we are  measuring time"
                      n4010 = call "timeInSeconds.vi"() -> ("Numeric"=w5392:dbl, "current time"=w5389:timestamp)  [unwired: 2 in]
                      n4011 = property on="current time" class="AbsTime (strict)"("Value"=w5389) -> ()  [unwired: 2 in, 2 out]
                      n4012 = Subtract(x=w5392, y=w5391) -> (x-y=w5390:dbl)
                      n4013 = Build Array (concatenate)(w5394, w5390) -> (w5393:dbl[])
                    }
                  }
                  n4014 = property on="data" class="Arr (strict)"("Value"=w5387) -> ()  [unwired: 2 in, 2 out]
                }
                frame #39 {
                  n4015 = local read "iPS_MagnetField"() -> (w5395:bool)
                  n4016 = property on="data" class="Arr (strict)"() -> ("Value"=w5396:dbl[])  [unwired: 2 in, 2 out]
                  n4017 = case shown="True" w5395 {
                    tunnel: w5396 -> [w5398 w5403]
                    tunnel: [w5398 w5402] -> w5397
                    frame False {
                      # "we are not Measuring magnetic field on IPS120-0"
                    }
                    frame True {
                      # "Measure magnetic field on Teslatron_iPS_Field"
                      n4018 = local read "iPS_addr_sweep"() -> (w5401:refnum<visa-resource-name>)
                      n4019 = call "iPSread.vi"("iPSreadCtrl"=iPSreadCtrl."MagnetField", "VISA resource name"=w5401) -> ("number"=w5400:dbl)  [unwired: 6 in, 3 out]
                      n4020 = Build Array (concatenate)(w5403, w5400) -> (w5402:dbl[])
                    }
                  }
                  n4021 = property on="data" class="Arr (strict)"("Value"=w5397) -> ()  [unwired: 2 in, 2 out]
                }
                frame #40 {
                  n4022 = property on="data" class="Arr (strict)"() -> ("Value"=w5405:dbl[])  [unwired: 2 in, 2 out]
                  n4023 = property on="Magnet_T" class="Bool (strict)"() -> ("Value"=w5404:bool)  [unwired: 2 in, 2 out]
                  n4024 = case shown="True" w5404 {
                    tunnel: w5405 -> [w5407 w5412]
                    tunnel: [w5407 w5411] -> w5406
                    frame False {
                      # "we are not Measuring magnetic field on IPS120-0"
                    }
                    frame True {
                      # "Measure magnetic_T on Teslatron"
                      n4025 = local read "iPS_addr_sweep"() -> (w5410:refnum<visa-resource-name>)
                      n4026 = call "iPSread.vi"("iPSreadCtrl"=iPSreadCtrl."Magnet Temp", "VISA resource name"=w5410) -> ("number"=w5409:dbl)  [unwired: 6 in, 3 out]
                      n4027 = Build Array (concatenate)(w5412, w5409) -> (w5411:dbl[])
                    }
                  }
                  n4028 = property on="data" class="Arr (strict)"("Value"=w5406) -> ()  [unwired: 2 in, 2 out]
                }
                frame #41 {
                  n4029 = property on="data" class="Arr (strict)"() -> ("Value"=w5414:dbl[])  [unwired: 2 in, 2 out]
                  n4030 = property on="SH_T" class="Bool (strict)"() -> ("Value"=w5413:bool)  [unwired: 2 in, 2 out]
                  n4031 = case shown="True" w5413 {
                    tunnel: w5414 -> [w5416 w5421]
                    tunnel: [w5416 w5420] -> w5415
                    frame False {
                      # "we are not Measuring magnetic field on IPS120-0"
                    }
                    frame True {
                      # "Measure  SH_T on Teslatron"
                      n4032 = local read "iPS_addr_sweep"() -> (w5419:refnum<visa-resource-name>)
                      n4033 = call "iPSread.vi"("iPSreadCtrl"=iPSreadCtrl."Switch Heater Temp", "VISA resource name"=w5419) -> ("number"=w5418:dbl)  [unwired: 6 in, 3 out]
                      n4034 = Build Array (concatenate)(w5421, w5418) -> (w5420:dbl[])
                    }
                  }
                  n4035 = property on="data" class="Arr (strict)"("Value"=w5415) -> ()  [unwired: 2 in, 2 out]
                }
                frame #42 {
                  # "check if current \non 2461 SouceMeter\nis to be measured"
                  n4036 = property on="data" class="Arr (strict)"() -> ("Value"=w5423:dbl[])  [unwired: 2 in, 2 out]
                  n4037 = property on="iTC_Sample_T" class="Bool (strict)"() -> ("Value"=w5422:bool)  [unwired: 2 in, 2 out]
                  n4038 = case shown="True" w5422 {
                    tunnel: w5423 -> [w5425 w5430]
                    tunnel: [w5425 w5429] -> w5424
                    frame False {
                      # "we are not measuring 2461, voltage (2461_meas_v)"
                    }
                    frame True {
                      # "we are  measuring 2461, voltage (2461_meas_v)"
                      n4039 = property on="iTC_addr_sweep" class="VISAName"() -> ("Value"=w5428:refnum<visa-resource-name>)  [unwired: 2 in, 2 out]
                      n4040 = call "iTCread.vi"("VISA resource name"=w5428, "iTCreadCtrl"=iTCreadCtrl."Sample Temp") -> ("number"=w5426:dbl)  [unwired: 5 in, 3 out]
                      n4041 = Build Array (concatenate)(w5430, w5426) -> (w5429:dbl[])
                    }
                  }
                  n4042 = property on="data" class="Arr (strict)"("Value"=w5424) -> ()  [unwired: 2 in, 2 out]
                }
                frame #43 {
                  # "check if current \non 2461 SouceMeter\nis to be measured"
                  n4043 = property on="data" class="Arr (strict)"() -> ("Value"=w5432:dbl[])  [unwired: 2 in, 2 out]
                  n4044 = property on="VTI_T" class="Bool (strict)"() -> ("Value"=w5431:bool)  [unwired: 2 in, 2 out]
                  n4045 = case shown="True" w5431 {
                    tunnel: w5432 -> [w5434 w5439]
                    tunnel: [w5434 w5438] -> w5433
                    frame False {
                      # "we are not measuring 2461, voltage (2461_meas_v)"
                    }
                    frame True {
                      # "we are  measuring 2461, voltage (2461_meas_v)"
                      n4046 = property on="iTC_addr_sweep" class="VISAName"() -> ("Value"=w5437:refnum<visa-resource-name>)  [unwired: 2 in, 2 out]
                      n4047 = call "iTCread.vi"("VISA resource name"=w5437, "iTCreadCtrl"=iTCreadCtrl."VTI Temp") -> ("number"=w5435:dbl)  [unwired: 5 in, 3 out]
                      n4048 = Build Array (concatenate)(w5439, w5435) -> (w5438:dbl[])
                    }
                  }
                  n4049 = property on="data" class="Arr (strict)"("Value"=w5433) -> ()  [unwired: 2 in, 2 out]
                }
                frame #44 {
                  # "check if current \non 2461 SouceMeter\nis to be measured"
                  n4050 = property on="data" class="Arr (strict)"() -> ("Value"=w5441:dbl[])  [unwired: 2 in, 2 out]
                  n4051 = property on="PT1_T" class="Bool (strict)"() -> ("Value"=w5440:bool)  [unwired: 2 in, 2 out]
                  n4052 = case shown="True" w5440 {
                    tunnel: w5441 -> [w5443 w5448]
                    tunnel: [w5443 w5447] -> w5442
                    frame False {
                      # "we are not measuring 2461, voltage (2461_meas_v)"
                    }
                    frame True {
                      # "we are  measuring 2461, voltage (2461_meas_v)"
                      n4053 = property on="iTC_addr_sweep" class="VISAName"() -> ("Value"=w5446:refnum<visa-resource-name>)  [unwired: 2 in, 2 out]
                      n4054 = call "iTCread.vi"("VISA resource name"=w5446, "iTCreadCtrl"=iTCreadCtrl."PT1 Temp") -> ("number"=w5444:dbl)  [unwired: 5 in, 3 out]
                      n4055 = Build Array (concatenate)(w5448, w5444) -> (w5447:dbl[])
                    }
                  }
                  n4056 = property on="data" class="Arr (strict)"("Value"=w5442) -> ()  [unwired: 2 in, 2 out]
                }
                frame #45 {
                  # "check if current \non 2461 SouceMeter\nis to be measured"
                  n4057 = property on="data" class="Arr (strict)"() -> ("Value"=w5450:dbl[])  [unwired: 2 in, 2 out]
                  n4058 = property on="PT2_T" class="Bool (strict)"() -> ("Value"=w5449:bool)  [unwired: 2 in, 2 out]
                  n4059 = case shown="True" w5449 {
                    tunnel: w5450 -> [w5452 w5457]
                    tunnel: [w5452 w5456] -> w5451
                    frame False {
                      # "we are not measuring 2461, voltage (2461_meas_v)"
                    }
                    frame True {
                      # "we are  measuring 2461, voltage (2461_meas_v)"
                      n4060 = property on="iTC_addr_sweep" class="VISAName"() -> ("Value"=w5455:refnum<visa-resource-name>)  [unwired: 2 in, 2 out]
                      n4061 = call "iTCread.vi"("VISA resource name"=w5455, "iTCreadCtrl"=iTCreadCtrl."PT2 Temp") -> ("number"=w5453:dbl)  [unwired: 5 in, 3 out]
                      n4062 = Build Array (concatenate)(w5457, w5453) -> (w5456:dbl[])
                    }
                  }
                  n4063 = property on="data" class="Arr (strict)"("Value"=w5451) -> ()  [unwired: 2 in, 2 out]
                }
                frame #46 {
                  # "check if current \non 2461 SouceMeter\nis to be measured"
                  n4064 = property on="data" class="Arr (strict)"() -> ("Value"=w5459:dbl[])  [unwired: 2 in, 2 out]
                  n4065 = property on="VTI_P" class="Bool (strict)"() -> ("Value"=w5458:bool)  [unwired: 2 in, 2 out]
                  n4066 = case shown="True" w5458 {
                    tunnel: w5459 -> [w5461 w5466]
                    tunnel: [w5461 w5465] -> w5460
                    frame False {
                      # "we are not measuring 2461, voltage (2461_meas_v)"
                    }
                    frame True {
                      # "we are  measuring 2461, voltage (2461_meas_v)"
                      n4067 = property on="iTC_addr_sweep" class="VISAName"() -> ("Value"=w5464:refnum<visa-resource-name>)  [unwired: 2 in, 2 out]
                      n4068 = call "iTCread.vi"("VISA resource name"=w5464, "iTCreadCtrl"=iTCreadCtrl."VTI Pressure") -> ("number"=w5462:dbl)  [unwired: 5 in, 3 out]
                      n4069 = Build Array (concatenate)(w5466, w5462) -> (w5465:dbl[])
                    }
                  }
                  n4070 = property on="data" class="Arr (strict)"("Value"=w5460) -> ()  [unwired: 2 in, 2 out]
                }
                frame #47 {
                  # "check if current \non 2461 SouceMeter\nis to be measured"
                  n4071 = property on="2461_meas_v" class="Bool (strict)"() -> ("Value"=w5467:bool)  [unwired: 2 in, 2 out]
                  n4072 = property on="data" class="Arr (strict)"() -> ("Value"=w5468:dbl[])  [unwired: 2 in, 2 out]
                  n4073 = case shown="True" w5467 {
                    tunnel: w5468 -> [w5470 w5475]
                    tunnel: [w5470 w5474] -> w5469
                    frame False {
                      # "we are not measuring 2461, voltage (2461_meas_v)"
                    }
                    frame True {
                      # "we are  measuring 2461, voltage (2461_meas_v)"
                      n4074 = property on="2461_addr_sweep" class="VISAName"() -> ("Value"=w5472:refnum<visa-resource-name>)  [unwired: 2 in, 2 out]
                      n4075 = call <instrlib>:"Read (Single Point).vi"("VISA resource name"=w5472) -> ("Data out"=w5471:string)  [unwired: 12 in, 2 out]
                      n4076 = Fract/Exp String To Number(string=w5471) -> (number=w5473:dbl)  [unwired: 3 in, 1 out]
                      n4077 = Build Array (concatenate)(w5475, w5473) -> (w5474:dbl[])
                    }
                  }
                  n4078 = property on="data" class="Arr (strict)"("Value"=w5469) -> ()  [unwired: 2 in, 2 out]
                }
                frame #48 {
                  # "check if current \non 2461 SouceMeter\nis to be measured"
                  n4079 = property on="2461_meas_i" class="Bool (strict)"() -> ("Value"=w5476:bool)  [unwired: 2 in, 2 out]
                  n4080 = property on="data" class="Arr (strict)"() -> ("Value"=w5477:dbl[])  [unwired: 2 in, 2 out]
                  n4081 = case shown="True" w5476 {
                    tunnel: w5477 -> [w5479 w5483]
                    tunnel: [w5479 w5482] -> w5478
                    frame False {
                      # "we are not measuring 2461, voltage (2461_meas_v)"
                    }
                    frame True {
                      # "we are  measuring 2461, curent (2461_meas_i)"
                      n4082 = property on="2461_addr_sweep" class="VISAName"() -> ("Value"=w5481:refnum<visa-resource-name>)  [unwired: 2 in, 2 out]
                      n4083 = call <instrlib>:"Get Source Level.vi"("VISA resource name"=w5481) -> ("Current Level Out"=w5480:dbl)  [unwired: 7 in, 3 out]
                      n4084 = Build Array (concatenate)(w5483, w5480) -> (w5482:dbl[])
                    }
                  }
                  n4085 = property on="data" class="Arr (strict)"("Value"=w5478) -> ()  [unwired: 2 in, 2 out]
                }
                frame #49 {
                  # "Record Step Value \nif it is mapping"
                  n4086 = property on="Step Loop" class="Bool (strict)"() -> ("Value"=w5485:bool)  [unwired: 2 in, 2 out]
                  n4087 = property on="data" class="Arr (strict)"() -> ("Value"=w5486:dbl[])  [unwired: 2 in, 2 out]
                  n4088 = case shown="True" w5485 {
                    tunnel: w5486 -> [w5487 w5490]
                    tunnel: [w5487 w5489] -> w5484
                    frame False {
                      # "We are not recording Step Value if it is linetrace"
                    }
                    frame True {
                      # "We are recording Step Value if it is mapping"
                      n4089 = property on="Current Step Value" class="DigNum (strict)"() -> ("Value"=w5488:dbl)  [unwired: 2 in, 2 out]
                      n4090 = Build Array (concatenate)(w5490, w5488) -> (w5489:dbl[])
                    }
                  }
                  n4091 = property on="data" class="Arr (strict)"("Value"=w5484) -> ()  [unwired: 2 in, 2 out]
                }
                frame #50 {
                  # "Record Step Value \nif it is mapping"
                  n4092 = property on="HyperLoop" class="Bool (strict)"() -> ("Value"=w5491:bool)  [unwired: 2 in, 2 out]
